vi "RT_stage_control_rev2.vi"() -> ()   [LabVIEW 2019]
uses:
  <vilib>/rvi/interface/nirviReadWriteControl/nirviReadWriteControl.xnode
  <vilib>/rvi/interface/nirviOpenFPGA/nirviOpenFPGA.xnode
  <vilib>/Platform/TimedLoop/XDataNode/XDataNode.xnode
  <vilib>/Platform/TimedLoop/XDataNode/nitl_modes.ctl
  <vilib>/Platform/TimedLoop/XDataNode/XDNodeRunTimeDep.lvlib
  <vilib>/Platform/TimedLoop/XDataNode/wakeup.ctl
  <vilib>/Platform/TimedLoop/XDataNode/timing_clust.ctl
  NiFpgaLv.dll
  <vilib>/Utility/error.llb/Error Cluster From Error Code.vi
  <vilib>/rvi/interface/Simulation/niFpgaSimulationCallBeginRW.vi
  <vilib>/rvi/errors/niLvFpgaAdjustHostInterfaceError.vi
  StageControl.ctl
  <vilib>/rvi/interface/nirviCloseFPGA/nirviCloseFPGA.xnode
  RasterControl.ctl
  <vilib>/FPGAPlugInAG/Dynamic/niLvFpga_Close_Dynamic.vi
  FPGA Bitfiles/studentchallenge_FPGATarget_FPGARADCWDAC3_gNVwU-DQYMc.lvbitx
  FPGA_R_ADC_W_DAC.vi
  <vilib>/FPGAPlugInAG/myRIO-1900/niLvFpga_Open_myRIO-1900.vi
  <vilib>/rvi/interface/common/dynamic/niFpgaDynamicAddResources.vi
panel:
  out "Late":i16
  in  "Return Speed":dbl=2.0 format="%#_13g"
  in  "Step Size [mm]":dbl=0.1 format="%#_13g"
  in  "tool up":bool
  in  "tool down":bool
  in  "Start":bool
  in  "Operation":T1
  out "FPGA Ref":refnum<k20>
  out "Raster Loop":T2
  out "Outer Loop":T1
  in  "Raster Width [mm]":dbl=6.0 format="%#_13g"
  in  "Velocity [mm/min]":dbl=100.0 format="%#_13g"
  in  "Stroke [mm]":dbl=6.0 format="%#_13g"
  in  "Zero Y":bool
  in  "Zero X":bool
  out "X Position":dbl format="%.4f"
  in  "Y Position [mm]":dbl format="%#_13g"
  in  "X Position [mm]":dbl format="%#_13g"
  out "Encoder B Offset":i32
  out "Encoder A Offset":i32
  out "Y Position":dbl format="%.4f"
  in  "stop":bool
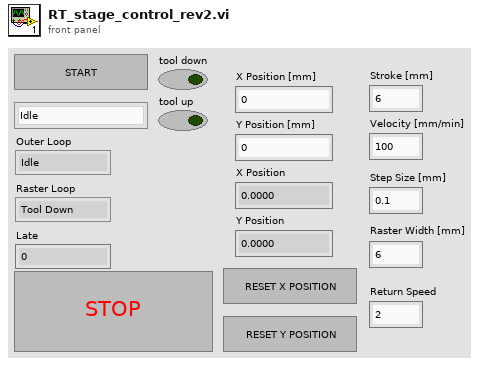
[diagram p1: front panel]
types:
  T1 = typedef "StageControl.ctl" = enum16{"Idle", "Raster", "Home X", "Home Y"}
  T2 = typedef "RasterControl.ctl" = enum16{"Tool Down", "Stroke", "Tool Up", "Return & Step"}
  T3 = typedef "XDNodeRunTimeDep.lvlib/timing_clust.ctl" = cluster{"Expected End [f-1]":u64, "Actual End [f-1]":u64, "Finished Late? [f-1]":bool, "Expected End [i-1]":u64, "Actual End [i-1]":u64, "Finished Late? [i-1]":bool, "Expected Start [i]":u64, "Actual Start [i]":u64, "Expected Start [f]":u64, "Actual Start [f]":u64, "Source Name":string, "Structure Name":string, "Period":i64, "Deadline":i64, "Offset":i64, "Start":i64, "Priority":i32, "Timeout":i32, "Mode":T4, "Wakeup Reason":T5, "Error":errorcluster, "Source Type":string, "Secondary Source Type":string, "Global End Time":u64, "Global Start Time":u64, "Frame Duration":u64, "Iteration Duration":u64, "Assigned CPU":i32, "I/O Scan Engine Mode":u32}
  T4 = typedef "XDNodeRunTimeDep.lvlib/nitl_modes.ctl" = enum32{"No Change", "Process missed periods, maintain original phase", "Discard missed periods, maintain original phase", "Process missed periods, ignore original phase", "Discard missed periods, ignore original phase"}
  T5 = typedef "XDNodeRunTimeDep.lvlib/wakeup.ctl" = enum32{"Normal", "Aborted", "Asynchronous wakeup", "Timing source error", "Timed loop error", "Timeout"}
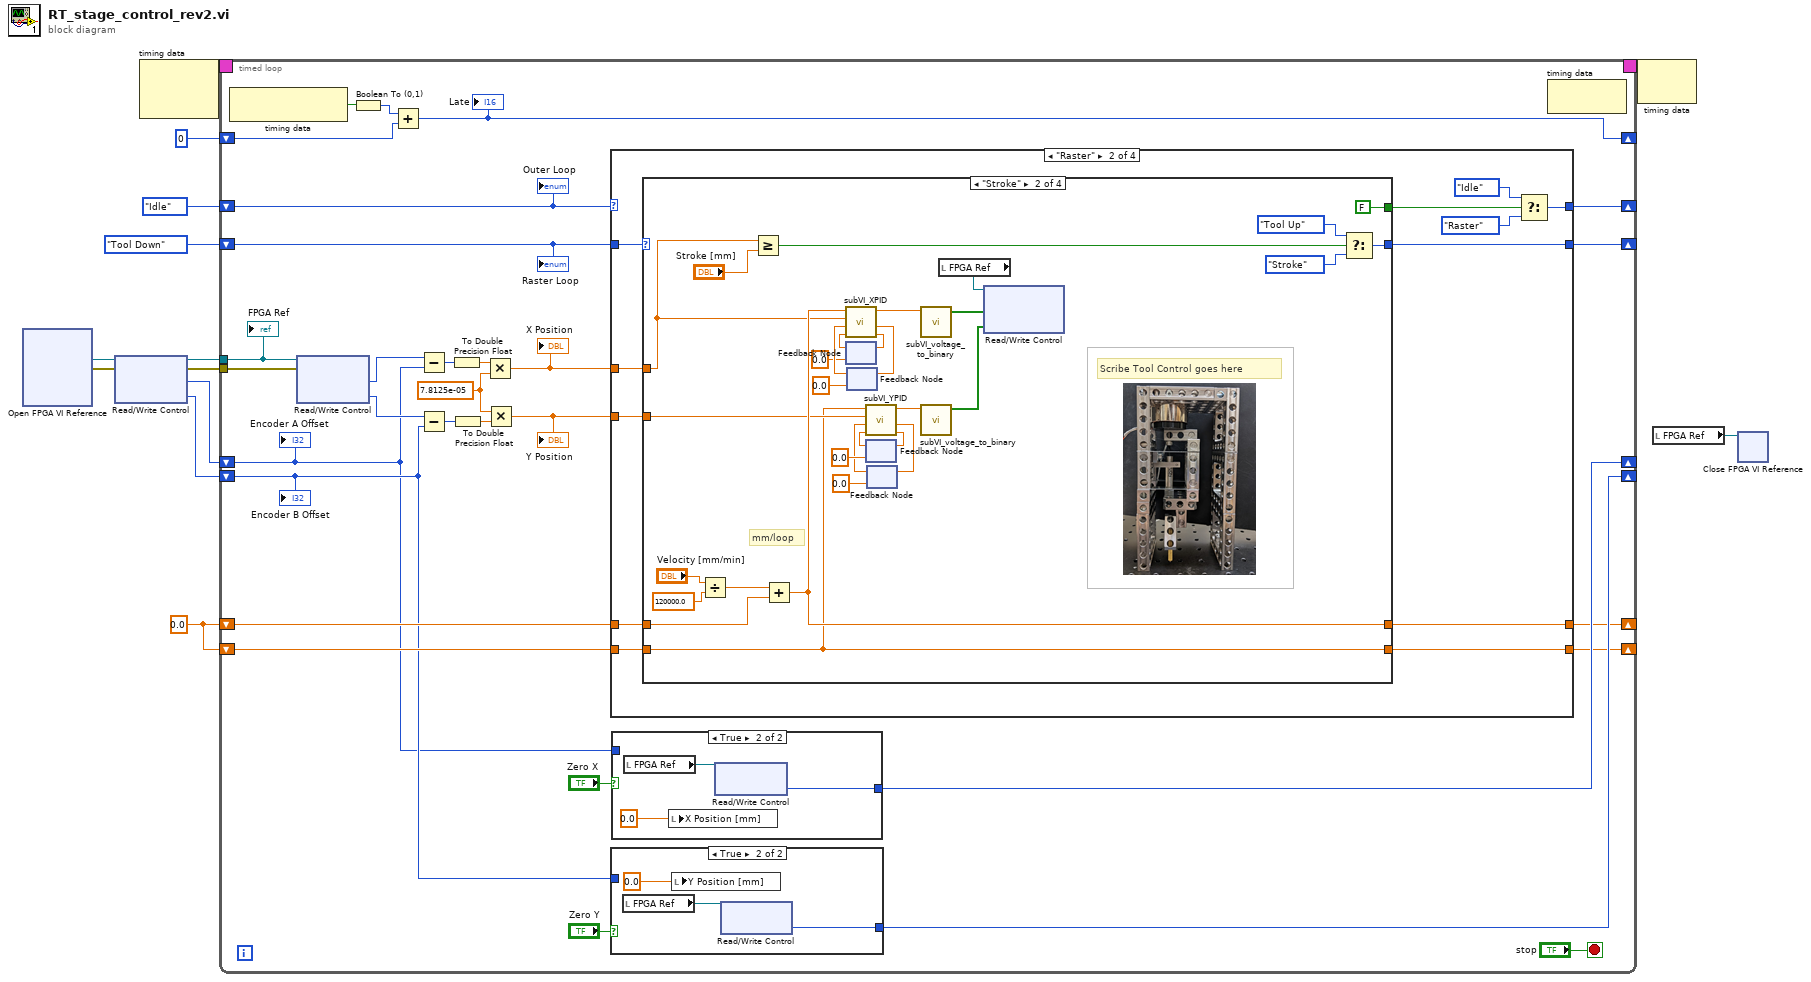
[diagram p0: block diagram]
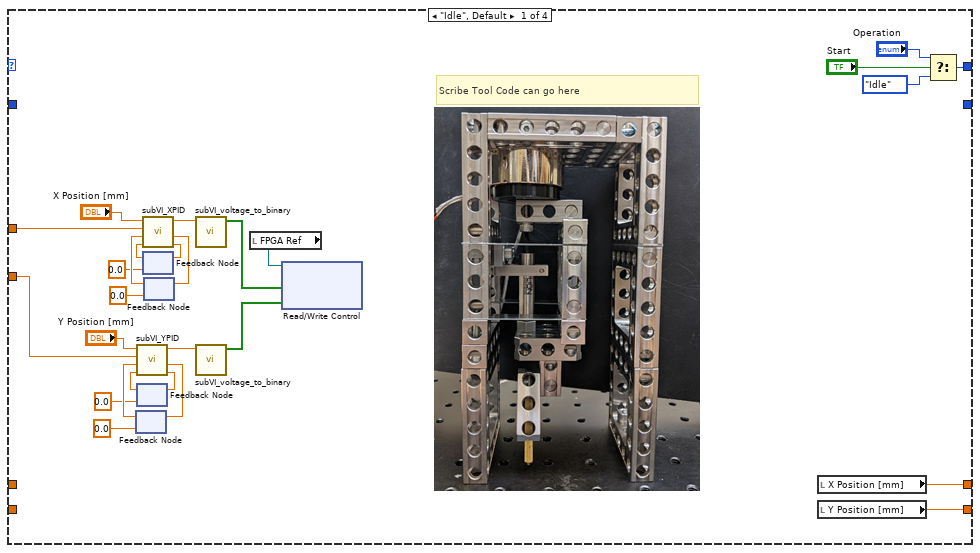
[diagram p2: hidden frame]
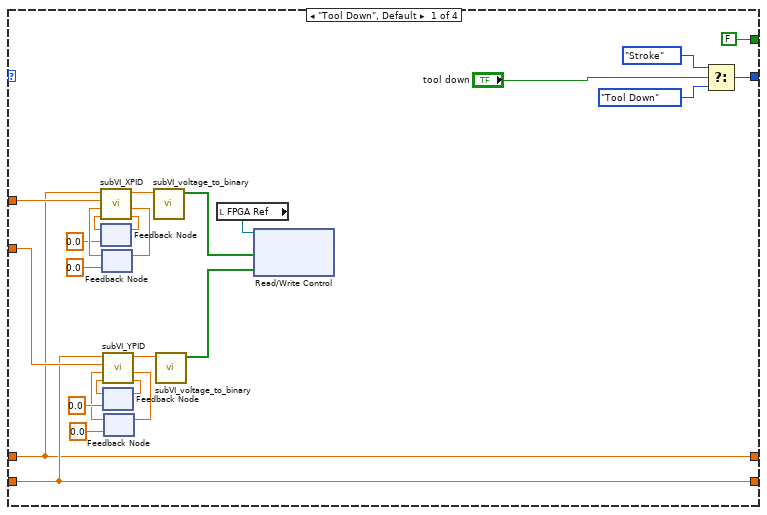
[diagram p3: hidden frame]
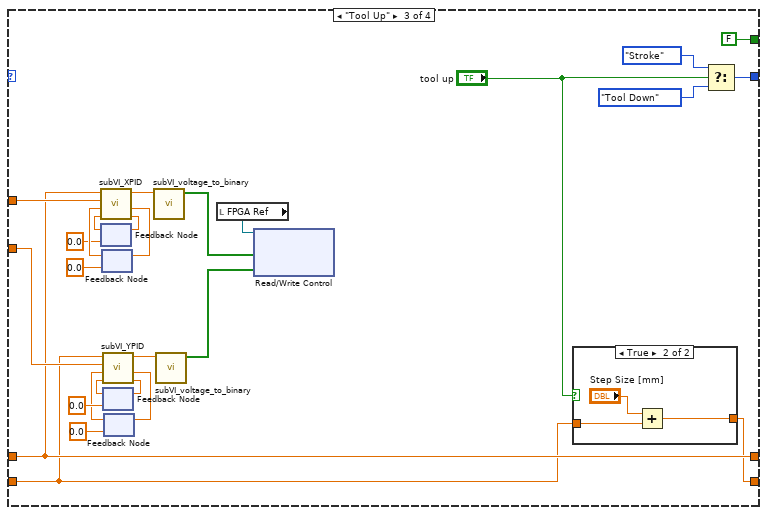
[diagram p4: hidden frame]
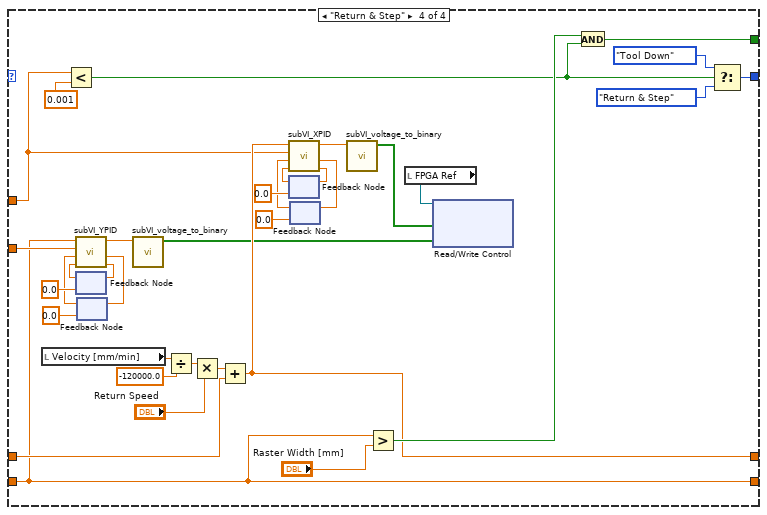
[diagram p6: hidden frame]
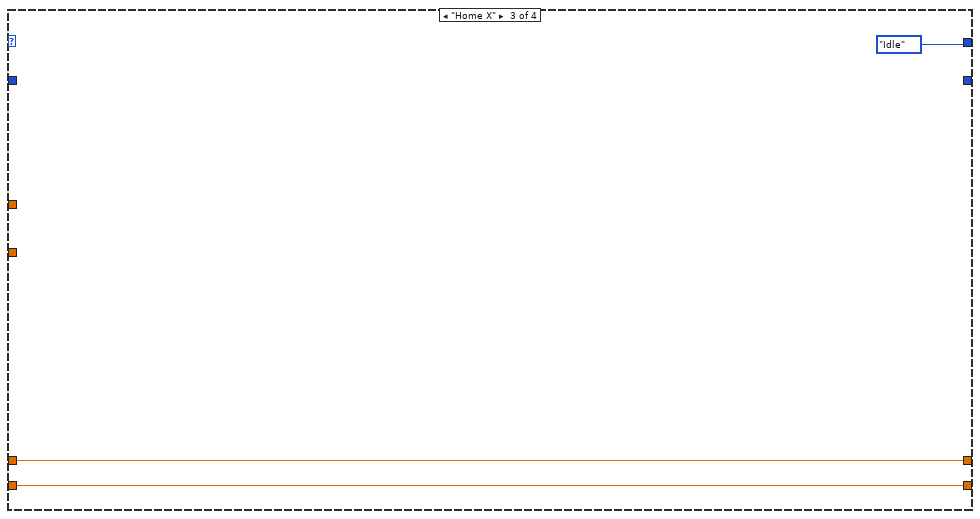
[diagram p7: hidden frame]
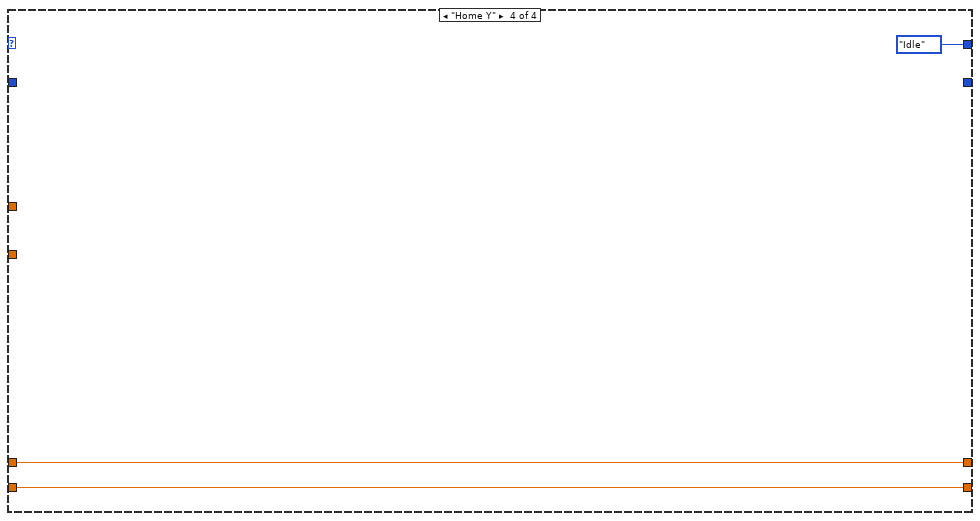
[diagram p8: hidden frame]
diagram:
  w3 = 0.0
  n1 = xnode "Open FPGA VI Reference"() -> ("FPGA VI Reference Out"=w11:refnum<k20>, "error out"=w10:errorcluster)  [unwired: 2 in]
  n2 = xnode "Read/Write Control"("FPGA VI Reference In"=w11, "error in"=w10) -> ("FPGA VI Reference Out"=w9:refnum<k20>, "error out"=w8:errorcluster, "Encoder A"=w7:i32, "Encoder B"=w6:i32)
  n3 = node-c288() -> (w13:T3)  [unwired: 2 in]
  n4 = timed-loop {
    shift-right: [w22] -> _
    shift-left: w7 -> [w23]
    timing: w13 -> [_]
    timing-out: [_] -> w12
    shift-right: [w21] -> _
    shift-left: w6 -> [w24]
    tunnel: w9 -> [w18]
    tunnel: w8 -> [w42]
    shift-right: [w34] -> _
    shift-left: StageControl."Idle" ("Enum 2") -> [w32]
    shift-right: [w29] -> _
    shift-left: RasterControl."Tool Down" -> [w30]
    shift-right: [w20] -> _
    shift-left: w3 -> [w28]
    shift-right: [w19] -> _
    shift-left: w3 -> [w27]
    shift-right: [w14] -> _
    shift-left: i16 0 -> [w15]
    stop <- "stop" stop-if-true
    w37 = 7.8125e-05 ("y")
    n5 = node-c288() -> (w17:bool)  [unwired: 1 in]
    n6 = xnode "Read/Write Control"("FPGA VI Reference In"=w18, "error in"=w42) -> ("Encoder A"=w36:i32, "Encoder B"=w35:i32)  [unwired: 2 out]
    n7 = Boolean To (0,1)(Boolean=w17) -> (0, 1=w16:i16)
    n8 = Add(x=w16, y=w15) -> (x+y=w14:i16)
    "Late" <- w14
    n9 = Subtract(x=w36, y=w23) -> (x-y=w40:i32)
    n10 = Subtract(x=w35, y=w24) -> (x-y=w39:i32)
    n11 = To Double Precision Float(number=w40) -> (double precision float=w41:dbl)
    n12 = To Double Precision Float(number=w39) -> (double precision float=w38:dbl)
    n13 = Multiply(x=w41, y=w37) -> (x*y=w31:dbl)
    "X Position" <- w31
    n14 = Multiply(x=w37, y=w38) -> (x*y=w33:dbl)
    "Y Position" <- w33
    n15 = case shown="\"Raster\"" w32 {
      tunnel: [w70 w81 StageControl."Idle" ("Enum 2") StageControl."Idle" ("Enum 2")] -> w34
      tunnel: w31 -> [w65 w76 _ _]
      tunnel: w33 -> [w64 w73 _ _]
      tunnel: w30 -> [_ w82 _ _]
      tunnel: [_ w77 _ _] -> w29
      tunnel: w28 -> [_ w75 w208 w210]
      tunnel: w27 -> [_ w74 w207 w209]
      tunnel: [w49 w72 w208 w210] -> w20
      tunnel: [w48 w71 w207 w209] -> w19
      frame "Idle", Default {
        # "Scribe Tool Code can go here"
        n16 = feedback #1(0.0 ("Error")) -> (w63:dbl)
        n17 = feedback #2(0.0 ("Cumulative Error Out")) -> (w61:dbl)
        n18 = call "subVI_YPID.vi"("Cumulative Error In"=w61, "Previous Error"=w63, "Encoder Position [mm]"=w64, "Desired Position [mm]"="Y Position [mm]") -> ("Cumulative Error Out"=w62:dbl, "Error"=w46:dbl, "Control Signal [V]"=w44:dbl)  [unwired: 5 in]
        n19 = feedback-in #1(w46) -> ()
        n20 = feedback-in #2(w62) -> ()
        n21 = feedback #3(0.0 ("Cumulative Error Out")) -> (w59:dbl)
        n22 = feedback #4(0.0 ("Error")) -> (w58:dbl)
        n23 = call "subVI_XPID.vi"("Cumulative Error In"=w59, "Previous Error"=w58, "Encoder Position [mm]"=w65, "Desired Position [mm]"="X Position [mm]") -> ("Cumulative Error Out"=w60:dbl, "Error"=w47:dbl, "Control Signal [V]"=w56:dbl)  [unwired: 5 in]
        n24 = feedback-in #3(w60) -> ()
        n25 = feedback-in #4(w47) -> ()
        n26 = call "subVI_voltage_to_binary.vi"("voltage"=w56) -> ("binary"=w55:bool[])  [unwired: 10 in]
        n27 = call "subVI_voltage_to_binary.vi"("voltage"=w44) -> ("binary"=w50:bool[])  [unwired: 10 in]
        n28 = local read "FPGA Ref"() -> (w45:refnum<k20>)
        n29 = xnode "Read/Write Control"("FPGA VI Reference In"=w45, "DAC 1 write"=w55, "DAC 2 write"=w50) -> ()  [unwired: 1 in, 2 out]
        n30 = local read "X Position [mm]"() -> (w49:dbl)
        n31 = local read "Y Position [mm]"() -> (w48:dbl)
        n32 = Select(t="Operation", s="Start", f=StageControl."Idle" ("Enum 2")) -> (s? t:f=w70:T1)
      }
      frame "Raster" {
        n33 = case shown="\"Stroke\"" w82 {
          tunnel: [FALSE FALSE FALSE w188] -> w78
          tunnel: [w107 w135 w165 w205] -> w77
          tunnel: w76 -> [w91 w109 w150 w174]
          tunnel: w75 -> [w88 w122 w147 w179]
          tunnel: w74 -> [w98 w112 w141 w171]
          tunnel: w73 -> [w99 w113 w157 w189]
          tunnel: [w88 w114 w147 w178] -> w72
          tunnel: [w98 w112 w140 w171] -> w71
          frame "Tool Down", Default {
            n34 = feedback #5(0.0 ("Cumulative Error Out")) -> (w95:dbl)
            n35 = feedback #6(0.0 ("Error")) -> (w94:dbl)
            n36 = call "subVI_XPID.vi"("Cumulative Error In"=w95, "Previous Error"=w94, "Encoder Position [mm]"=w91, "Desired Position [mm]"=w88) -> ("Cumulative Error Out"=w96:dbl, "Error"=w86:dbl, "Control Signal [V]"=w97:dbl)  [unwired: 5 in]
            n37 = feedback-in #5(w96) -> ()
            n38 = feedback-in #6(w86) -> ()
            n39 = feedback #7(0.0 ("Cumulative Error Out")) -> (w101:dbl)
            n40 = feedback #8(0.0 ("Error")) -> (w102:dbl)
            n41 = call "subVI_YPID.vi"("Cumulative Error In"=w101, "Previous Error"=w102, "Encoder Position [mm]"=w99, "Desired Position [mm]"=w98) -> ("Cumulative Error Out"=w100:dbl, "Error"=w87:dbl, "Control Signal [V]"=w83:dbl)  [unwired: 5 in]
            n42 = feedback-in #7(w100) -> ()
            n43 = feedback-in #8(w87) -> ()
            n44 = call "subVI_voltage_to_binary.vi"("voltage"=w97) -> ("binary"=w90:bool[])  [unwired: 10 in]
            n45 = call "subVI_voltage_to_binary.vi"("voltage"=w83) -> ("binary"=w89:bool[])  [unwired: 10 in]
            n46 = local read "FPGA Ref"() -> (w84:refnum<k20>)
            n47 = xnode "Read/Write Control"("FPGA VI Reference In"=w84, "DAC 1 write"=w90, "DAC 2 write"=w89) -> ()  [unwired: 1 in, 2 out]
            n48 = Select(t=RasterControl."Stroke", s="tool down", f=RasterControl."Tool Down") -> (s? t:f=w107:T2)
          }
          frame "Stroke" {
            # "Scribe Tool Control goes here"
            # "mm/loop"
            n49 = Divide(x="Velocity [mm/min]", y=120000.0) -> (x/y=w131:dbl)
            n50 = Greater Or Equal?(x=w109, y="Stroke [mm]") -> (x >= y?=w133:bool)
            n51 = Add(x=w131, y=w122) -> (x+y=w114:dbl)
            n52 = feedback #9(0.0 ("Cumulative Error Out")) -> (w118:dbl)
            n53 = feedback #10(0.0 ("Error")) -> (w117:dbl)
            n54 = call "subVI_XPID.vi"("Cumulative Error In"=w118, "Previous Error"=w117, "Encoder Position [mm]"=w109, "Desired Position [mm]"=w114) -> ("Cumulative Error Out"=w119:dbl, "Error"=w120:dbl, "Control Signal [V]"=w121:dbl)  [unwired: 5 in]
            n55 = feedback-in #9(w119) -> ()
            n56 = feedback-in #10(w120) -> ()
            n57 = feedback #11(0.0 ("Cumulative Error Out")) -> (w126:dbl)
            n58 = feedback #12(0.0 ("Error")) -> (w127:dbl)
            n59 = call "subVI_YPID.vi"("Cumulative Error In"=w126, "Previous Error"=w127, "Encoder Position [mm]"=w113, "Desired Position [mm]"=w112) -> ("Cumulative Error Out"=w125:dbl, "Error"=w124:dbl, "Control Signal [V]"=w123:dbl)  [unwired: 5 in]
            n60 = feedback-in #11(w125) -> ()
            n61 = feedback-in #12(w124) -> ()
            n62 = call "subVI_voltage_to_binary.vi"("voltage"=w121) -> ("binary"=w111:bool[])  [unwired: 10 in]
            n63 = call "subVI_voltage_to_binary.vi"("voltage"=w123) -> ("binary"=w110:bool[])  [unwired: 10 in]
            n64 = local read "FPGA Ref"() -> (w130:refnum<k20>)
            n65 = xnode "Read/Write Control"("FPGA VI Reference In"=w130, "DAC 1 write"=w111, "DAC 2 write"=w110) -> ()  [unwired: 1 in, 2 out]
            n66 = Select(t=RasterControl."Tool Up", s=w133, f=RasterControl."Stroke") -> (s? t:f=w135:T2)
          }
          frame "Tool Up" {
            n67 = feedback #13(0.0 ("Cumulative Error Out")) -> (w154:dbl)
            n68 = feedback #14(0.0 ("Error")) -> (w153:dbl)
            n69 = call "subVI_XPID.vi"("Cumulative Error In"=w154, "Previous Error"=w153, "Encoder Position [mm]"=w150, "Desired Position [mm]"=w147) -> ("Cumulative Error Out"=w155:dbl, "Error"=w145:dbl, "Control Signal [V]"=w156:dbl)  [unwired: 5 in]
            n70 = feedback-in #13(w155) -> ()
            n71 = feedback-in #14(w145) -> ()
            n72 = feedback #15(0.0 ("Cumulative Error Out")) -> (w159:dbl)
            n73 = feedback #16(0.0 ("Error")) -> (w160:dbl)
            n74 = call "subVI_YPID.vi"("Cumulative Error In"=w159, "Previous Error"=w160, "Encoder Position [mm]"=w157, "Desired Position [mm]"=w141) -> ("Cumulative Error Out"=w158:dbl, "Error"=w146:dbl, "Control Signal [V]"=w143:dbl)  [unwired: 5 in]
            n75 = feedback-in #15(w158) -> ()
            n76 = feedback-in #16(w146) -> ()
            n77 = call "subVI_voltage_to_binary.vi"("voltage"=w156) -> ("binary"=w149:bool[])  [unwired: 10 in]
            n78 = call "subVI_voltage_to_binary.vi"("voltage"=w143) -> ("binary"=w148:bool[])  [unwired: 10 in]
            n79 = local read "FPGA Ref"() -> (w144:refnum<k20>)
            n80 = xnode "Read/Write Control"("FPGA VI Reference In"=w144, "DAC 1 write"=w149, "DAC 2 write"=w148) -> ()  [unwired: 1 in, 2 out]
            n81 = case shown="True" "tool up" {
              tunnel: w141 -> [w167 w169]
              tunnel: [w167 w170] -> w140
              frame False {
              }
              frame True {
                n82 = Add(x="Step Size [mm]", y=w169) -> (x+y=w170:dbl)
              }
            }
            n83 = Select(t=RasterControl."Stroke", s="tool up", f=RasterControl."Tool Down") -> (s? t:f=w165:T2)
          }
          frame "Return & Step" {
            n84 = local read "Velocity [mm/min]"() -> (w184:dbl)
            n85 = Less?(x=w174, y=0.001) -> (x < y?=w173:bool)
            n86 = feedback #17(0.0 ("Cumulative Error Out")) -> (w192:dbl)
            n87 = feedback #18(0.0 ("Error")) -> (w193:dbl)
            n88 = call "subVI_YPID.vi"("Cumulative Error In"=w192, "Previous Error"=w193, "Encoder Position [mm]"=w189, "Desired Position [mm]"=w171) -> ("Cumulative Error Out"=w191:dbl, "Error"=w190:dbl, "Control Signal [V]"=w185:dbl)  [unwired: 5 in]
            n89 = feedback-in #17(w191) -> ()
            n90 = feedback-in #18(w190) -> ()
            n91 = call "subVI_voltage_to_binary.vi"("voltage"=w185) -> ("binary"=w177:bool[])  [unwired: 10 in]
            n92 = Divide(x=w184, y=-120000.0) -> (x/y=w182:dbl)
            n93 = Multiply(x=w182, y="Return Speed") -> (x*y=w180:dbl)
            n94 = Add(x=w180, y=w179) -> (x+y=w178:dbl)
            n95 = feedback #19(0.0 ("Cumulative Error Out")) -> (w198:dbl)
            n96 = feedback #20(0.0 ("Error")) -> (w199:dbl)
            n97 = call "subVI_XPID.vi"("Cumulative Error In"=w198, "Previous Error"=w199, "Encoder Position [mm]"=w174, "Desired Position [mm]"=w178) -> ("Cumulative Error Out"=w197:dbl, "Error"=w196:dbl, "Control Signal [V]"=w186:dbl)  [unwired: 5 in]
            n98 = feedback-in #19(w197) -> ()
            n99 = feedback-in #20(w196) -> ()
            n100 = call "subVI_voltage_to_binary.vi"("voltage"=w186) -> ("binary"=w176:bool[])  [unwired: 10 in]
            n101 = Greater?(x=w171, y="Raster Width [mm]") -> (0:w187:bool)
            n102 = local read "FPGA Ref"() -> (w202:refnum<k20>)
            n103 = xnode "Read/Write Control"("FPGA VI Reference In"=w202, "DAC 1 write"=w176, "DAC 2 write"=w177) -> ()  [unwired: 1 in, 2 out]
            n104 = And(x=w187, y=w173) -> (x .and. y?=w188:bool)
            n105 = Select(t=RasterControl."Tool Down", s=w173, f=RasterControl."Return & Step") -> (s? t:f=w205:T2)
          }
        }
        n106 = Select(t=StageControl."Idle" ("Enum 2"), s=w78, f=StageControl."Raster" ("Enum 2")) -> (s? t:f=w81:T1)
      }
      frame "Home X" {
      }
      frame "Home Y" {
      }
    }
    n107 = case shown="True" "Zero Y" {
      tunnel: w24 -> [w215 _]
      tunnel: [w215 w217] -> w21
      frame False {
      }
      frame True {
        n108 = local read "FPGA Ref"() -> (w216:refnum<k20>)
        n109 = local write "Y Position [mm]"(0.0 ("Y Relative Position [mm]")) -> ()
        n110 = xnode "Read/Write Control"("FPGA VI Reference In"=w216) -> ("Encoder B"=w217:i32)  [unwired: 1 in, 2 out]
      }
    }
    n111 = case shown="True" "Zero X" {
      tunnel: w23 -> [w219 _]
      tunnel: [w219 w221] -> w22
      frame False {
      }
      frame True {
        n112 = local read "FPGA Ref"() -> (w220:refnum<k20>)
        n113 = local write "X Position [mm]"(0.0 ("X Relative Position [mm]")) -> ()
        n114 = xnode "Read/Write Control"("FPGA VI Reference In"=w220) -> ("Encoder A"=w221:i32)  [unwired: 1 in, 2 out]
      }
    }
    n115 = node-c288() -> ()  [unwired: 1 in, 1 out]
    "Encoder A Offset" <- w23
    "Encoder B Offset" <- w24
    "Outer Loop" <- w32
    "Raster Loop" <- w30
    "FPGA Ref" <- w18
  }
  n116 = node-c288(w12) -> ()  [unwired: 1 out]
  n117 = local read "FPGA Ref"() -> (w2:refnum<k20>)
  n118 = xnode "Close FPGA VI Reference"("FPGA VI Reference In"=w2) -> ()  [unwired: 1 in, 1 out]
